vi "read e-series file names.vi"(3 "error in (no error)":errorcluster, 5 "INI File":string) -> (0 "error out":errorcluster, 2 "E-Series File Names":string[](array[string]))   [LabVIEW 2018, in "CSV Series Read.lvlib"]
uses:
  CSV Series Read.lvlib
  <vilib>/Utility/config.llb/Read Key (String).vi
  <vilib>/Utility/config.llb/NI_LVConfig.lvlib
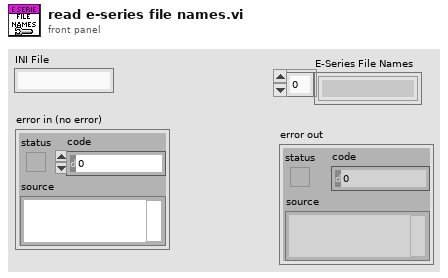
[diagram p1: front panel]
types:
  T1 = typedef "NI_LVConfig.lvlib/Config Data RefNum.ctl" = refnum<k1>
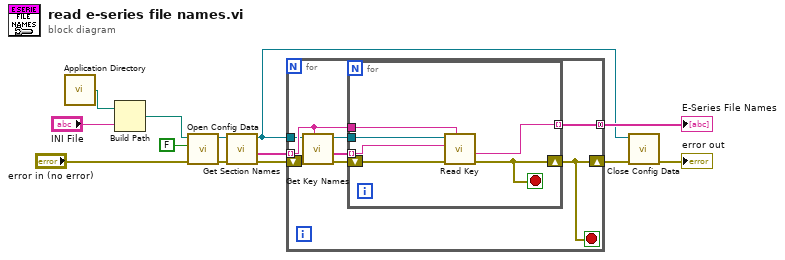
[diagram p0: block diagram]
diagram:
  n1 = call <vilib>:"Application Directory.vi"() -> ("Application Directory"=w13:path)
  n2 = Build Path(base path=w13, name or relative path="INI File") -> (appended path=w10:path)
  n3 = call <vilib>:"Open Config Data.vi"("error in (no error)"="error in (no error)", "create file if necessary (T)"=FALSE, "configuration file path"=w10) -> ("error out"=w8:errorcluster, "refnum"=w7:T1)  [unwired: 6 in, 1 out]
  n4 = call <vilib>:"Get Section Names.vi"("error in (no error)"=w8, "refnum"=w7) -> ("error out"=w5:errorcluster, "section names"=w6:string[], "refnum out"=w3:T1)  [unwired: 7 in]
  n5 = for {
    tunnel: w3 -> [w14]
    tunnel: w6 -> [w18] mode=indexing
    shift-right: [w16] -> w2
    shift-left: w5 -> [w21]
    tunnel: [w17] -> w4 mode=concatenating
    stop <- w16 stop-if-true
    n6 = call <vilib>:"Get Key Names.vi"("section"=w18, "error in (no error)"=w21, "refnum"=w14) -> ("error out"=w20:errorcluster, "key names"=w19:string[], "refnum out"=w15:T1)  [unwired: 5 in, 1 out]
    n7 = for {
      shift-right: [w23] -> w16
      shift-left: w20 -> [w27]
      tunnel: w19 -> [w26] mode=indexing
      tunnel: w18 -> [w25]
      tunnel: [w24] -> w17 mode=indexing
      tunnel: w15 -> [w22]
      stop <- w23 stop-if-true
      n8 = call-poly <vilib>:"Read Key.vi"("section"=w25, "error in (no error)"=w27, "key"=w26, "refnum"=w22) -> ("error out"=w23:errorcluster, "value"=w24:string)  [unwired: 4 in, 2 out]
    }
  }
  "E-Series File Names" <- w4
  n9 = call <vilib>:"Close Config Data.vi"("error in (no error)"=w2, "refnum"=w3) -> ("error out"=→"error out":errorcluster)  [unwired: 8 in, 1 out]
